vi "HandleObservationSync_003.vi"(8 "error in (no error)":errorcluster, 11 "S4GUI in":refnum<class "S4GUI.lvclass">) -> (0 "error out":errorcluster, 3 "S4GUI out":refnum<class "S4GUI.lvclass">)   [LabVIEW 2018, in "S4GUI.lvclass"] (continued)
          n1276 = call "Read connection.vi"("error in (no error)"=w3469, "Server in"=w3471) -> ("error out"=w3497:errorcluster, "connection"=w3481:bool, "Server out"=w3498:refnum<class "Acquisition.lvclass">)  [unwired: 7 in]
          n1277 = And(x=w3481, y=w3459) -> (x .and. y?=w3482:bool)
          n1278 = case shown="True" w3482 {
            tunnel: w3498 -> [w3607 w3623]
            tunnel: w3497 -> [w3606 w3622]
            tunnel: [w3607 w3620] -> w3515
            tunnel: [w3606 w3619] -> w3513
            tunnel: [w3603 u32 0 ("New_State")] -> w3488
            tunnel: w3459 -> [w3602 _]
            frame False {
              n1279 = Select(t=u32 2, s=w3602, f=u32 0) -> (s? t:f=w3603:u32)
            }
            frame True {
              n1280 = call-dynamic "Read Channel.vi"("error in (no error)"=w3622, "Acquisition in"=w3623) -> ("error out"=w3615:errorcluster, "Channel.lvclass"=w3614:refnum<class "Channel.lvclass">, "Acquisition out"=w3621:refnum<class "Acquisition.lvclass">)  [unwired: 7 in]
              n1281 = call-dynamic "Read State Machine.vi"("error in (no error)"=w3615, "Device in"=w3614) -> ("error out"=w3616:errorcluster, "State Machine.lvclass"=w3618:refnum<class "State Machine.lvclass">, "Device out"=w3612:refnum<class "Channel.lvclass">)  [unwired: 7 in]
              n1282 = call "Next State.vi"("error in (no error)"=w3616, "New_State"=50, "State Machine in"=w3618) -> ("error out"=w3609:errorcluster, "State Machine out"=w3610:refnum<class "State Machine.lvclass">)  [unwired: 7 in]
              n1283 = call-dynamic "Write State Machine.vi"("error in (no error)"=w3609, "State Machine.lvclass"=w3610, "Device in"=w3612) -> ("error out"=w3611:errorcluster, "Device out"=w3613:refnum<class "Channel.lvclass">)  [unwired: 7 in]
              n1284 = call-dynamic "Write Channel.vi"("error in (no error)"=w3611, "Channel.lvclass"=w3613, "Acquisition in"=w3621) -> ("error out"=w3619:errorcluster, "Acquisition out"=w3620:refnum<class "Acquisition.lvclass">)  [unwired: 7 in]
            }
          }
          n1285 = call "Write AcquisitionB.vi"("error in (no error)"=w3513, "Acquisition.lvclass"=w3515, "S4ACS_GUI in"=w3514) -> ("error out"=w3509:errorcluster, "S4ACS_GUI out"=w3508:refnum<class "S4GUI.lvclass">)  [unwired: 7 in]
          n1286 = call-dynamic "Read AcquisitionC.vi"("error in (no error)"=w3509, "S4ACS_GUI in"=w3508) -> ("error out"=w3466:errorcluster, "Acquisition.lvclass"=w3468:refnum<class "Acquisition.lvclass">, "S4ACS_GUI out"=w3511:refnum<class "S4GUI.lvclass">)  [unwired: 7 in]
          n1287 = call-dynamic "Read enabled.vi"("error in (no error)"=w3466, "Server in"=w3468) -> ("error out"=w3465:errorcluster, "enabled"=w3458:bool, "Server out"=w3467:refnum<class "Acquisition.lvclass">)  [unwired: 7 in]
          n1288 = call "Read connection.vi"("error in (no error)"=w3465, "Server in"=w3467) -> ("error out"=w3495:errorcluster, "connection"=w3478:bool, "Server out"=w3496:refnum<class "Acquisition.lvclass">)  [unwired: 7 in]
          n1289 = And(x=w3478, y=w3458) -> (x .and. y?=w3480:bool)
          n1290 = case shown="True" w3480 {
            tunnel: [w3584 w3593] -> w3512
            tunnel: [w3585 w3592] -> w3510
            tunnel: w3496 -> [w3585 w3590]
            tunnel: w3495 -> [w3584 w3589]
            tunnel: [w3581 u32 0 ("New_State")] -> w3487
            tunnel: w3458 -> [w3580 _]
            frame False {
              n1291 = Select(t=u32 4, s=w3580, f=u32 0) -> (s? t:f=w3581:u32)
            }
            frame True {
              n1292 = call-dynamic "Read Channel.vi"("error in (no error)"=w3589, "Acquisition in"=w3590) -> ("error out"=w3597:errorcluster, "Channel.lvclass"=w3598:refnum<class "Channel.lvclass">, "Acquisition out"=w3591:refnum<class "Acquisition.lvclass">)  [unwired: 7 in]
              n1293 = call-dynamic "Read State Machine.vi"("error in (no error)"=w3597, "Device in"=w3598) -> ("error out"=w3596:errorcluster, "State Machine.lvclass"=w3594:refnum<class "State Machine.lvclass">, "Device out"=w3600:refnum<class "Channel.lvclass">)  [unwired: 7 in]
              n1294 = call "Next State.vi"("error in (no error)"=w3596, "New_State"=50, "State Machine in"=w3594) -> ("error out"=w3588:errorcluster, "State Machine out"=w3587:refnum<class "State Machine.lvclass">)  [unwired: 7 in]
              n1295 = call-dynamic "Write State Machine.vi"("error in (no error)"=w3588, "State Machine.lvclass"=w3587, "Device in"=w3600) -> ("error out"=w3601:errorcluster, "Device out"=w3599:refnum<class "Channel.lvclass">)  [unwired: 7 in]
              n1296 = call-dynamic "Write Channel.vi"("error in (no error)"=w3601, "Channel.lvclass"=w3599, "Acquisition in"=w3591) -> ("error out"=w3593:errorcluster, "Acquisition out"=w3592:refnum<class "Acquisition.lvclass">)  [unwired: 7 in]
            }
          }
          n1297 = call-dynamic "Write AcquisitionC.vi"("error in (no error)"=w3512, "Acquisition.lvclass"=w3510, "S4ACS_GUI in"=w3511) -> ("error out"=w3506:errorcluster, "S4ACS_GUI out"=w3505:refnum<class "S4GUI.lvclass">)  [unwired: 7 in]
          n1298 = call-dynamic "Read AcquisitionD.vi"("error in (no error)"=w3506, "S4ACS_GUI in"=w3505) -> ("error out"=w3462:errorcluster, "Acquisition.lvclass"=w3464:refnum<class "Acquisition.lvclass">, "S4ACS_GUI out"=w3504:refnum<class "S4GUI.lvclass">)  [unwired: 7 in]
          n1299 = call-dynamic "Read enabled.vi"("error in (no error)"=w3462, "Server in"=w3464) -> ("error out"=w3461:errorcluster, "enabled"=w3457:bool, "Server out"=w3463:refnum<class "Acquisition.lvclass">)  [unwired: 7 in]
          n1300 = call "Read connection.vi"("error in (no error)"=w3461, "Server in"=w3463) -> ("error out"=w3493:errorcluster, "connection"=w3477:bool, "Server out"=w3494:refnum<class "Acquisition.lvclass">)  [unwired: 7 in]
          n1301 = And(x=w3477, y=w3457) -> (x .and. y?=w3479:bool)
          n1302 = case shown="True" w3479 {
            tunnel: w3493 -> [w3562 w3579]
            tunnel: [w3562 w3578] -> w3507
            tunnel: w3494 -> [w3563 w3569]
            tunnel: [w3563 w3567] -> w3503
            tunnel: [w3559 u32 0 ("New_State")] -> w3486
            tunnel: w3457 -> [w3558 _]
            frame False {
              n1303 = Select(t=u32 8, s=w3558, f=u32 0) -> (s? t:f=w3559:u32)
            }
            frame True {
              n1304 = call-dynamic "Read Channel.vi"("error in (no error)"=w3579, "Acquisition in"=w3569) -> ("error out"=w3574:errorcluster, "Channel.lvclass"=w3573:refnum<class "Channel.lvclass">, "Acquisition out"=w3568:refnum<class "Acquisition.lvclass">)  [unwired: 7 in]
              n1305 = call-dynamic "Read State Machine.vi"("error in (no error)"=w3574, "Device in"=w3573) -> ("error out"=w3575:errorcluster, "State Machine.lvclass"=w3577:refnum<class "State Machine.lvclass">, "Device out"=w3571:refnum<class "Channel.lvclass">)  [unwired: 7 in]
              n1306 = call "Next State.vi"("error in (no error)"=w3575, "New_State"=50, "State Machine in"=w3577) -> ("error out"=w3565:errorcluster, "State Machine out"=w3566:refnum<class "State Machine.lvclass">)  [unwired: 7 in]
              n1307 = call-dynamic "Write State Machine.vi"("error in (no error)"=w3565, "State Machine.lvclass"=w3566, "Device in"=w3571) -> ("error out"=w3570:errorcluster, "Device out"=w3572:refnum<class "Channel.lvclass">)  [unwired: 7 in]
              n1308 = call-dynamic "Write Channel.vi"("error in (no error)"=w3570, "Channel.lvclass"=w3572, "Acquisition in"=w3568) -> ("error out"=w3578:errorcluster, "Acquisition out"=w3567:refnum<class "Acquisition.lvclass">)  [unwired: 7 in]
            }
          }
          n1309 = call-dynamic "Write AcquisitionD.vi"("error in (no error)"=w3507, "Acquisition.lvclass"=w3503, "S4ACS_GUI in"=w3504) -> ("error out"=w3502:errorcluster, "S4ACS_GUI out"=w3501:refnum<class "S4GUI.lvclass">)  [unwired: 7 in]
          n1310 = Compound Arithmetic op=ADD(w3489, w3488, w3487, w3486) -> (w3490:u32)
          n1311 = case shown="0, Default" w3490 {
            tunnel: w3485 -> [w3527 _ _ _ _ _ _ _ _ _ _ _ _ _ _ _]
            tunnel: [w3526 u32 1 ("Obs_state") u32 1 ("Obs_state") u32 1 ("Obs_state") u32 1 ("Obs_state") u32 1 ("Obs_state") u32 1 ("Obs_state") u32 1 ("Obs_state") u32 1 ("Obs_state") u32 1 ("Obs_state") u32 1 ("Obs_state") u32 1 ("Obs_state") u32 1 ("Obs_state") u32 1 ("Obs_state") u32 1 ("Obs_state") u32 1 ("Obs_state")] -> w3491
            tunnel: ["" ("Error Msg") "ERROR: Lost channel 1 connection... - HandleObservationSync.vi state 323" ("Error Msg") "ERROR: Lost channel 2 connection...- HandleObservationSync.vi state 323" ("Error Msg") "ERROR: Lost channels 1 and 2 connection...- HandleObservationSync.vi state 323" ("Error Msg") "ERROR: Lost channel 3 connection...- HandleObservationSync.vi state 323" ("Error Msg") "ERROR: Lost channels 1 and  3 connection...- HandleObservationSync.vi state 323" ("Error Msg") "ERROR:  Lost channels 2 and  3 connection...- HandleObservationSync.vi state 323" ("Error Msg") "ERROR:  Lost channels 1, 2 and  3 connection...- HandleObservationSync.vi state 323" ("Error Msg") "ERROR: Lost channel 4 connection...- HandleObservationSync.vi state 323" ("Error Msg") "ERROR:  Lost channels 1 and 4 connection...- HandleObservationSync.vi state 323" ("Error Msg") "ERROR:  Lost channels 2 and 4 connection...- HandleObservationSync.vi state 323" ("Error Msg") "ERROR: Lost channels 1, 2 and 4 connection...- HandleObservationSync.vi state 323" ("Error Msg") "ERROR: Lost channels 3 and 4 connection...- HandleObservationSync.vi state 323" ("Error Msg") "ERROR: Lost channels 1, 3 and 4 connection...- HandleObservationSync.vi state 323" ("Error Msg") "ERROR: Lost channels 2, 3 and 4 connection...- HandleObservationSync.vi state 323" ("Error Msg") "ERROR: Lost channels 1, 2, 3 and 4 connection...- HandleObservationSync.vi state 323" ("Error Msg")] -> w3492
            frame 0, Default {
              n1312 = Increment(x=w3527) -> (x+1=w3526:u32)
              n1313 = Tick Count (ms)() -> (millisecond timer value=w3524:u32)
              n1314 = local write "time1"(w3524) -> ()
            }
            frame 1 {
            }
            frame 2 {
            }
            frame 3 {
            }
            frame 4 {
            }
            frame 5 {
            }
            frame 6 {
            }
            frame 7 {
            }
            frame 8 {
            }
            frame 9 {
            }
            frame 10 {
            }
            frame 11 {
            }
            frame 12 {
            }
            frame 13 {
            }
            frame 14 {
            }
            frame 15 {
            }
          }
          n1315 = Bundle By Name(cluster=w3501, "Obs_state"=w3491, "Error Msg"=w3492) -> (w3518:refnum<class "S4GUI.lvclass">)
        }
        frame 324 {
          # "Espera terminar a execução do comando atual \nantes de ir ao proximo passo da Observação."
          n1316 = call-dynamic "Read AcquisitionA.vi"("error in (no error)"=w3699, "S4ACS_GUI in"=w3700) -> ("error out"=w3681:errorcluster, "Acquisition.lvclass"=w3682:refnum<class "Acquisition.lvclass">, "S4ACS_GUI out"=w3702:refnum<class "S4GUI.lvclass">)  [unwired: 7 in]
          n1317 = call "Read connection.vi"("error in (no error)"=w3681, "Server in"=w3682) -> ("error out"=w3680:errorcluster, "connection"=w3679:bool, "Server out"=w3678:refnum<class "Acquisition.lvclass">)  [unwired: 7 in]
          n1318 = case shown="True" w3679 {
            tunnel: w3680 -> [w3811 w3832]
            tunnel: [w3812 w3830] -> w3703
            tunnel: [w3811 w3829] -> w3701
            tunnel: [TRUE w3818] -> w3660
            tunnel: w3678 -> [w3812 w3821]
            tunnel: [FALSE w3813] -> w3658
            frame False {
            }
            frame True {
              n1319 = call-dynamic "Read Channel.vi"("error in (no error)"=w3832, "Acquisition in"=w3821) -> ("error out"=w3815:errorcluster, "Channel.lvclass"=w3817:refnum<class "Channel.lvclass">, "Acquisition out"=w3831:refnum<class "Acquisition.lvclass">)  [unwired: 7 in]
              n1320 = call-dynamic "Read wait_expose.vi"("error in (no error)"=w3815, "Channel in"=w3817) -> ("error out"=w3814:errorcluster, "wait_expose"=w3813:bool, "Channel out"=w3816:refnum<class "Channel.lvclass">)  [unwired: 7 in]
              n1321 = call-dynamic "Read State Machine.vi"("error in (no error)"=w3814, "Device in"=w3816) -> ("error out"=w3823:errorcluster, "State Machine.lvclass"=w3825:refnum<class "State Machine.lvclass">, "Device out"=w3827:refnum<class "Channel.lvclass">)  [unwired: 7 in]
              n1322 = call-dynamic "Read State.vi"("error in (no error)"=w3823, "State Machine in"=w3825) -> ("error out"=w3822:errorcluster, "State"=w3819:i32, "State Machine out"=w3824:refnum<class "State Machine.lvclass">)  [unwired: 7 in]
              n1323 = Greater?(x=w3819, y=53 ("x")) -> (0:w3818:bool)
              n1324 = call-dynamic "Write State Machine.vi"("error in (no error)"=w3822, "State Machine.lvclass"=w3824, "Device in"=w3827) -> ("error out"=w3826:errorcluster, "Device out"=w3828:refnum<class "Channel.lvclass">)  [unwired: 7 in]
              n1325 = call-dynamic "Write Channel.vi"("error in (no error)"=w3826, "Channel.lvclass"=w3828, "Acquisition in"=w3831) -> ("error out"=w3829:errorcluster, "Acquisition out"=w3830:refnum<class "Acquisition.lvclass">)  [unwired: 7 in]
            }
          }
          n1326 = call-dynamic "Write AcquisitionA.vi"("error in (no error)"=w3701, "Acquisition.lvclass"=w3703, "S4ACS_GUI in"=w3702) -> ("error out"=w3696:errorcluster, "S4ACS_GUI out"=w3695:refnum<class "S4GUI.lvclass">)  [unwired: 7 in]
          n1327 = call "Read AcquisitionB.vi"("error in (no error)"=w3696, "S4ACS_GUI in"=w3695) -> ("error out"=w3673:errorcluster, "Acquisition.lvclass"=w3677:refnum<class "Acquisition.lvclass">, "S4ACS_GUI out"=w3697:refnum<class "S4GUI.lvclass">)  [unwired: 7 in]
          n1328 = call "Read connection.vi"("error in (no error)"=w3673, "Server in"=w3677) -> ("error out"=w3674:errorcluster, "connection"=w3675:bool, "Server out"=w3676:refnum<class "Acquisition.lvclass">)  [unwired: 7 in]
          n1329 = case shown="True" w3675 {
            tunnel: w3674 -> [w3787 w3800]
            tunnel: w3676 -> [w3788 w3799]
            tunnel: [TRUE w3794] -> w3662
            tunnel: [w3787 w3798] -> w3694
            tunnel: [w3788 w3797] -> w3693
            tunnel: [FALSE w3789] -> w3657
            frame False {
            }
            frame True {
              n1330 = call-dynamic "Read Channel.vi"("error in (no error)"=w3800, "Acquisition in"=w3799) -> ("error out"=w3791:errorcluster, "Channel.lvclass"=w3793:refnum<class "Channel.lvclass">, "Acquisition out"=w3801:refnum<class "Acquisition.lvclass">)  [unwired: 7 in]
              n1331 = call-dynamic "Read wait_expose.vi"("error in (no error)"=w3791, "Channel in"=w3793) -> ("error out"=w3790:errorcluster, "wait_expose"=w3789:bool, "Channel out"=w3792:refnum<class "Channel.lvclass">)  [unwired: 7 in]
              n1332 = call-dynamic "Read State Machine.vi"("error in (no error)"=w3790, "Device in"=w3792) -> ("error out"=w3807:errorcluster, "State Machine.lvclass"=w3805:refnum<class "State Machine.lvclass">, "Device out"=w3803:refnum<class "Channel.lvclass">)  [unwired: 7 in]
              n1333 = call-dynamic "Read State.vi"("error in (no error)"=w3807, "State Machine in"=w3805) -> ("error out"=w3808:errorcluster, "State"=w3796:i32, "State Machine out"=w3806:refnum<class "State Machine.lvclass">)  [unwired: 7 in]
              n1334 = Greater?(x=w3796, y=53 ("x")) -> (0:w3794:bool)
              n1335 = call-dynamic "Write State Machine.vi"("error in (no error)"=w3808, "State Machine.lvclass"=w3806, "Device in"=w3803) -> ("error out"=w3804:errorcluster, "Device out"=w3802:refnum<class "Channel.lvclass">)  [unwired: 7 in]
              n1336 = call-dynamic "Write Channel.vi"("error in (no error)"=w3804, "Channel.lvclass"=w3802, "Acquisition in"=w3801) -> ("error out"=w3798:errorcluster, "Acquisition out"=w3797:refnum<class "Acquisition.lvclass">)  [unwired: 7 in]
            }
          }
          n1337 = call "Write AcquisitionB.vi"("error in (no error)"=w3694, "Acquisition.lvclass"=w3693, "S4ACS_GUI in"=w3697) -> ("error out"=w3686:errorcluster, "S4ACS_GUI out"=w3685:refnum<class "S4GUI.lvclass">)  [unwired: 7 in]
          n1338 = call-dynamic "Read AcquisitionC.vi"("error in (no error)"=w3686, "S4ACS_GUI in"=w3685) -> ("error out"=w3669:errorcluster, "Acquisition.lvclass"=w3672:refnum<class "Acquisition.lvclass">, "S4ACS_GUI out"=w3688:refnum<class "S4GUI.lvclass">)  [unwired: 7 in]
          n1339 = call "Read connection.vi"("error in (no error)"=w3669, "Server in"=w3672) -> ("error out"=w3668:errorcluster, "connection"=w3670:bool, "Server out"=w3671:refnum<class "Acquisition.lvclass">)  [unwired: 7 in]
          n1340 = case shown="True" w3670 {
            tunnel: [w3763 w3777] -> w3689
            tunnel: [w3764 w3776] -> w3687
            tunnel: w3668 -> [w3763 w3773]
            tunnel: w3671 -> [w3764 w3774]
            tunnel: [TRUE w3770] -> w3661
            tunnel: [FALSE w3765] -> w3656
            frame False {
            }
            frame True {
              n1341 = call-dynamic "Read Channel.vi"("error in (no error)"=w3773, "Acquisition in"=w3774) -> ("error out"=w3767:errorcluster, "Channel.lvclass"=w3769:refnum<class "Channel.lvclass">, "Acquisition out"=w3775:refnum<class "Acquisition.lvclass">)  [unwired: 7 in]
              n1342 = call-dynamic "Read wait_expose.vi"("error in (no error)"=w3767, "Channel in"=w3769) -> ("error out"=w3766:errorcluster, "wait_expose"=w3765:bool, "Channel out"=w3768:refnum<class "Channel.lvclass">)  [unwired: 7 in]
              n1343 = call-dynamic "Read State Machine.vi"("error in (no error)"=w3766, "Device in"=w3768) -> ("error out"=w3783:errorcluster, "State Machine.lvclass"=w3781:refnum<class "State Machine.lvclass">, "Device out"=w3779:refnum<class "Channel.lvclass">)  [unwired: 7 in]
              n1344 = call-dynamic "Read State.vi"("error in (no error)"=w3783, "State Machine in"=w3781) -> ("error out"=w3784:errorcluster, "State"=w3771:i32, "State Machine out"=w3782:refnum<class "State Machine.lvclass">)  [unwired: 7 in]
              n1345 = Greater?(x=w3771, y=53 ("x")) -> (0:w3770:bool)
              n1346 = call-dynamic "Write State Machine.vi"("error in (no error)"=w3784, "State Machine.lvclass"=w3782, "Device in"=w3779) -> ("error out"=w3780:errorcluster, "Device out"=w3778:refnum<class "Channel.lvclass">)  [unwired: 7 in]
              n1347 = call-dynamic "Write Channel.vi"("error in (no error)"=w3780, "Channel.lvclass"=w3778, "Acquisition in"=w3775) -> ("error out"=w3777:errorcluster, "Acquisition out"=w3776:refnum<class "Acquisition.lvclass">)  [unwired: 7 in]
            }
          }
          n1348 = call-dynamic "Write AcquisitionC.vi"("error in (no error)"=w3689, "Acquisition.lvclass"=w3687, "S4ACS_GUI in"=w3688) -> ("error out"=w3683:errorcluster, "S4ACS_GUI out"=w3684:refnum<class "S4GUI.lvclass">)  [unwired: 7 in]
          n1349 = call-dynamic "Read AcquisitionD.vi"("error in (no error)"=w3683, "S4ACS_GUI in"=w3684) -> ("error out"=w3664:errorcluster, "Acquisition.lvclass"=w3667:refnum<class "Acquisition.lvclass">, "S4ACS_GUI out"=w3690:refnum<class "S4GUI.lvclass">)  [unwired: 7 in]
          n1350 = call "Read connection.vi"("error in (no error)"=w3664, "Server in"=w3667) -> ("error out"=w3663:errorcluster, "connection"=w3665:bool, "Server out"=w3666:refnum<class "Acquisition.lvclass">)  [unwired: 7 in]
          n1351 = case shown="True" w3665 {
            tunnel: [w3740 w3760] -> w3692
            tunnel: [w3739 w3759] -> w3691
            tunnel: w3666 -> [w3740 w3758]
            tunnel: w3663 -> [w3739 w3757]
            tunnel: [TRUE w3746] -> w3659
            tunnel: [FALSE w3741] -> w3655
            frame False {
            }
            frame True {
              n1352 = call-dynamic "Read Channel.vi"("error in (no error)"=w3757, "Acquisition in"=w3758) -> ("error out"=w3743:errorcluster, "Channel.lvclass"=w3745:refnum<class "Channel.lvclass">, "Acquisition out"=w3756:refnum<class "Acquisition.lvclass">)  [unwired: 7 in]
              n1353 = call-dynamic "Read wait_expose.vi"("error in (no error)"=w3743, "Channel in"=w3745) -> ("error out"=w3742:errorcluster, "wait_expose"=w3741:bool, "Channel out"=w3744:refnum<class "Channel.lvclass">)  [unwired: 7 in]
              n1354 = call-dynamic "Read State Machine.vi"("error in (no error)"=w3742, "Device in"=w3744) -> ("error out"=w3750:errorcluster, "State Machine.lvclass"=w3752:refnum<class "State Machine.lvclass">, "Device out"=w3754:refnum<class "Channel.lvclass">)  [unwired: 7 in]
              n1355 = call-dynamic "Read State.vi"("error in (no error)"=w3750, "State Machine in"=w3752) -> ("error out"=w3749:errorcluster, "State"=w3747:i32, "State Machine out"=w3751:refnum<class "State Machine.lvclass">)  [unwired: 7 in]
              n1356 = Greater?(x=w3747, y=53 ("x")) -> (0:w3746:bool)
              n1357 = call-dynamic "Write State Machine.vi"("error in (no error)"=w3749, "State Machine.lvclass"=w3751, "Device in"=w3754) -> ("error out"=w3753:errorcluster, "Device out"=w3755:refnum<class "Channel.lvclass">)  [unwired: 7 in]
              n1358 = call-dynamic "Write Channel.vi"("error in (no error)"=w3753, "Channel.lvclass"=w3755, "Acquisition in"=w3756) -> ("error out"=w3759:errorcluster, "Acquisition out"=w3760:refnum<class "Acquisition.lvclass">)  [unwired: 7 in]
            }
          }
          n1359 = call-dynamic "Write AcquisitionD.vi"("error in (no error)"=w3691, "Acquisition.lvclass"=w3692, "S4ACS_GUI in"=w3690) -> ("error out"=w3647:errorcluster, "S4ACS_GUI out"=w3650:refnum<class "S4GUI.lvclass">)  [unwired: 7 in]
          n1360 = Compound Arithmetic op=AND(w3660, w3662, w3661, w3659) -> (w3654:bool)
          n1361 = Compound Arithmetic op=OR(w3658, w3657, w3656, w3655) -> (w3652:bool)
          n1362 = call-dynamic "VerifErrors.vi"("error in (no error)"=w3647, "S4GUI in"=w3650) -> ("error out"=w3646:errorcluster, "Error value"=w3649:u32, "S4GUI out"=w3648:refnum<class "S4GUI.lvclass">)  [unwired: 7 in]
          n1363 = case shown="False" w3654 {
            tunnel: w3648 -> [w3706 w3736]
            tunnel: [w3712 w3735] -> w3651
            tunnel: w3653 -> [_ w3734]
            tunnel: w3652 -> [_ w3730]
            tunnel: w3649 -> [w3704 _]
            frame False {
              # "Aguardando iniciar exposição por 5s"
              n1364 = Tick Count (ms)() -> (millisecond timer value=w3711:u32)
              n1365 = local read "time1"() -> (w3705:u32)
              n1366 = Subtract(x=w3711, y=w3705) -> (x-y=w3708:u32)
              n1367 = To Double Precision Float(number=w3708) -> (double precision float=w3710:dbl)
              n1368 = Less?(x=5000.0 ("y"), y=w3710) -> (x < y?=w3709:bool)
              n1369 = case shown="False" w3709 {
                tunnel: w3706 -> [w3715 w3728]
                tunnel: [w3713 w3727] -> w3712
                tunnel: w3704 -> [w3714 _]
                frame False {
                  n1370 = case shown="1..15" w3714 {
                    selector: w3714 -> [_ w3723]
                    tunnel: [w3716 w3718] -> w3713
                    tunnel: w3715 -> [w3716 w3724]
                    frame 0, Default {
                    }
                    frame 1..15 {
                      n1371 = Number To Decimal String(number=w3723) -> (decimal integer string=w3720:string)  [unwired: 1 in]
                      n1372 = Concatenate Strings("CHANNEL ERROR <", w3720, ">: Error flag TRUE - see ACS panel.  HandleObservationSync.vi - state 324.") -> (w3722:string)
                      n1373 = Bundle By Name(cluster=w3724, "Obs_state"=u32 1, "Error Msg"=w3722) -> (w3718:refnum<class "S4GUI.lvclass">)
                    }
                  }
                }
                frame True {
                  n1374 = Bundle By Name(cluster=w3728, "Obs_state"=u32 1, "Error Msg"="ERROR: Acquisition Timeout. HandleObservationSync.vi - state 324.") -> (w3727:refnum<class "S4GUI.lvclass">)
                }
              }
            }
            frame True {
              # "327: Verifica incremento de ciclo."
              # "Iniciou aquisição..."
              n1375 = Increment(x=w3734) -> (x+1=w3731:u32)
              n1376 = Select(t=u32 327, s=w3730, f=w3731) -> (s? t:f=w3729:u32)
              n1377 = Tick Count (ms)() -> (millisecond timer value=w3733:u32)
              n1378 = Bundle By Name(cluster=w3736, "Obs_state"=w3729) -> (w3735:refnum<class "S4GUI.lvclass">)
              n1379 = local write "time307"(w3733) -> ()
            }
          }
          n1380 = Bundle By Name(cluster=w3651, "mode EXPOSE"=w3652) -> (w3698:refnum<class "S4GUI.lvclass">)
        }
        frame 325 {
          n1381 = Unbundle By Name(w3842) -> ("mode EXPOSE"=w3841:bool)
          n1382 = case shown="True" w3841 {
            tunnel: w3842 -> [w3895 w3962]
            tunnel: w3847 -> [w3894 w3961]
            tunnel: [w3893 w3959] -> w3846
            tunnel: [w3892 w3960] -> w3845
            tunnel: [w3891 w3958] -> w3835
            tunnel: w3843 -> [w3883 w3958]
            tunnel: [w3882 w3923] -> w3840
            tunnel: [w3882 w3922] -> w3839
            tunnel: [w3882 w3921] -> w3838
            tunnel: [w3882 w3920] -> w3837
            frame False {
              w3882 = 0
              n1383 = call-dynamic "Read Sync Box.lvclass.vi"("error in (no error)"=w3894, "SPARC4_AC in"=w3895) -> ("error out"=w3888:errorcluster, "Sync Box.lvclass"=w3890:refnum<class "Sync Box.lvclass">, "SPARC4_AC out"=w3885:refnum<class "S4GUI.lvclass">)  [unwired: 7 in]
              n1384 = call "Read connection.vi"("error in (no error)"=w3888, "Server in"=w3890) -> ("error out"=w3887:errorcluster, "connection"=w3886:bool, "Server out"=w3889:refnum<class "Sync Box.lvclass">)  [unwired: 7 in]
              n1385 = case shown="True" w3886 {
                tunnel: w3887 -> [w3901 w3919]
                tunnel: [w3902 w3917] -> w3897
                tunnel: [w3901 w3904] -> w3896
                tunnel: w3883 -> [w3898 w3903]
                tunnel: [w3900 w3903] -> w3891
                tunnel: w3889 -> [w3902 w3908]
                tunnel: w3885 -> [w3899 w3905]
                tunnel: [w3899 w3905] -> w3884
                frame False {
                  n1386 = Increment(x=w3898) -> (x+1=w3900:u32)
                }
                frame True {
                  # "Envia comando FIRE para o SyncBox"
                  n1387 = call-dynamic "Read Trigger.lvclass.vi"("error in (no error)"=w3919, "Sync Box in"=w3908) -> ("error out"=w3913:errorcluster, "Trigger.lvclass"=w3912:refnum<class "Trigger.lvclass">, "Sync Box out"=w3918:refnum<class "Sync Box.lvclass">)  [unwired: 7 in]
                  n1388 = call-dynamic "Read State Machine.vi"("error in (no error)"=w3913, "Device in"=w3912) -> ("error out"=w3914:errorcluster, "State Machine.lvclass"=w3916:refnum<class "State Machine.lvclass">, "Device out"=w3910:refnum<class "Trigger.lvclass">)  [unwired: 7 in]
                  n1389 = call "Next State.vi"("error in (no error)"=w3914, "New_State"=40, "State Machine in"=w3916) -> ("error out"=w3906:errorcluster, "State Machine out"=w3907:refnum<class "State Machine.lvclass">)  [unwired: 7 in]
                  n1390 = call-dynamic "Write State Machine.vi"("error in (no error)"=w3906, "State Machine.lvclass"=w3907, "Device in"=w3910) -> ("error out"=w3909:errorcluster, "Device out"=w3911:refnum<class "Trigger.lvclass">)  [unwired: 7 in]
                  n1391 = call-dynamic "Write Trigger.lvclass.vi"("error in (no error)"=w3909, "Trigger.lvclass"=w3911, "Sync Box in"=w3918) -> ("error out"=w3904:errorcluster, "Sync Box out"=w3917:refnum<class "Sync Box.lvclass">)  [unwired: 7 in]
                }
              }
              n1392 = call-dynamic "Write Sync Box.lvclass.vi"("error in (no error)"=w3896, "Sync Box.lvclass"=w3897, "SPARC4_AC in"=w3884) -> ("error out"=w3893:errorcluster, "SPARC4_AC out"=w3892:refnum<class "S4GUI.lvclass">)  [unwired: 7 in]
            }
            frame True {
              # "Envia comando EXPOSE para os canais ativos"
              n1393 = call-dynamic "Read AcquisitionA.vi"("error in (no error)"=w3961, "S4ACS_GUI in"=w3962) -> ("error out"=w3955:errorcluster, "Acquisition.lvclass"=w3957:refnum<class "Acquisition.lvclass">, "S4ACS_GUI out"=w3981:refnum<class "S4GUI.lvclass">)  [unwired: 7 in]
              n1394 = call-dynamic "Read enabled.vi"("error in (no error)"=w3955, "Server in"=w3957) -> ("error out"=w3954:errorcluster, "enabled"=w3927:bool, "Server out"=w3956:refnum<class "Acquisition.lvclass">)  [unwired: 7 in]
              n1395 = call "Read connection.vi"("error in (no error)"=w3954, "Server in"=w3956) -> ("error out"=w3963:errorcluster, "connection"=w3952:bool, "Server out"=w3964:refnum<class "Acquisition.lvclass">)  [unwired: 7 in]
              n1396 = And(x=w3952, y=w3927) -> (x .and. y?=w3953:bool)
              n1397 = case shown="True" w3953 {
                tunnel: w3964 -> [w4054 w4070]
                tunnel: w3963 -> [w4053 w4069]
                tunnel: [w4054 w4067] -> w3982
                tunnel: [w4053 w4066] -> w3980
                tunnel: [w4049 0] -> w3923
                tunnel: w3927 -> [w4050 _]
                frame False {
                  n1398 = Select(t=1, s=w4050, f=0) -> (s? t:f=w4049:i32)
                }
                frame True {
                  n1399 = call-dynamic "Read Channel.vi"("error in (no error)"=w4069, "Acquisition in"=w4070) -> ("error out"=w4062:errorcluster, "Channel.lvclass"=w4061:refnum<class "Channel.lvclass">, "Acquisition out"=w4068:refnum<class "Acquisition.lvclass">)  [unwired: 7 in]
                  n1400 = call-dynamic "Read State Machine.vi"("error in (no error)"=w4062, "Device in"=w4061) -> ("error out"=w4063:errorcluster, "State Machine.lvclass"=w4065:refnum<class "State Machine.lvclass">, "Device out"=w4059:refnum<class "Channel.lvclass">)  [unwired: 7 in]
                  n1401 = call "Next State.vi"("error in (no error)"=w4063, "New_State"=50, "State Machine in"=w4065) -> ("error out"=w4056:errorcluster, "State Machine out"=w4057:refnum<class "State Machine.lvclass">)  [unwired: 7 in]
                  n1402 = call-dynamic "Write State Machine.vi"("error in (no error)"=w4056, "State Machine.lvclass"=w4057, "Device in"=w4059) -> ("error out"=w4058:errorcluster, "Device out"=w4060:refnum<class "Channel.lvclass">)  [unwired: 7 in]
                  n1403 = call-dynamic "Write Channel.vi"("error in (no error)"=w4058, "Channel.lvclass"=w4060, "Acquisition in"=w4068) -> ("error out"=w4066:errorcluster, "Acquisition out"=w4067:refnum<class "Acquisition.lvclass">)  [unwired: 7 in]
                }
              }
              n1404 = call-dynamic "Write AcquisitionA.vi"("error in (no error)"=w3980, "Acquisition.lvclass"=w3982, "S4ACS_GUI in"=w3981) -> ("error out"=w3978:errorcluster, "S4ACS_GUI out"=w3979:refnum<class "S4GUI.lvclass">)  [unwired: 7 in]
              n1405 = call "Read AcquisitionB.vi"("error in (no error)"=w3978, "S4ACS_GUI in"=w3979) -> ("error out"=w3946:errorcluster, "Acquisition.lvclass"=w3948:refnum<class "Acquisition.lvclass">, "S4ACS_GUI out"=w3976:refnum<class "S4GUI.lvclass">)  [unwired: 7 in]
              n1406 = call-dynamic "Read enabled.vi"("error in (no error)"=w3946, "Server in"=w3948) -> ("error out"=w3950:errorcluster, "enabled"=w3926:bool, "Server out"=w3951:refnum<class "Acquisition.lvclass">)  [unwired: 7 in]
              n1407 = call "Read connection.vi"("error in (no error)"=w3950, "Server in"=w3951) -> ("error out"=w3945:errorcluster, "connection"=w3949:bool, "Server out"=w3947:refnum<class "Acquisition.lvclass">)  [unwired: 7 in]
              n1408 = And(x=w3949, y=w3926) -> (x .and. y?=w3944:bool)
              n1409 = case shown="False" w3944 {
                tunnel: w3947 -> [w4032 w4048]
                tunnel: w3945 -> [w4031 w4047]
                tunnel: [w4032 w4045] -> w3977
                tunnel: [w4031 w4044] -> w3975
                tunnel: [w4028 0] -> w3922
                tunnel: w3926 -> [w4027 _]
                frame False {
                  n1410 = Select(t=2, s=w4027, f=0) -> (s? t:f=w4028:i32)
                }
                frame True {
                  n1411 = call-dynamic "Read Channel.vi"("error in (no error)"=w4047, "Acquisition in"=w4048) -> ("error out"=w4040:errorcluster, "Channel.lvclass"=w4039:refnum<class "Channel.lvclass">, "Acquisition out"=w4046:refnum<class "Acquisition.lvclass">)  [unwired: 7 in]
                  n1412 = call-dynamic "Read State Machine.vi"("error in (no error)"=w4040, "Device in"=w4039) -> ("error out"=w4041:errorcluster, "State Machine.lvclass"=w4043:refnum<class "State Machine.lvclass">, "Device out"=w4037:refnum<class "Channel.lvclass">)  [unwired: 7 in]
                  n1413 = call "Next State.vi"("error in (no error)"=w4041, "New_State"=50, "State Machine in"=w4043) -> ("error out"=w4034:errorcluster, "State Machine out"=w4035:refnum<class "State Machine.lvclass">)  [unwired: 7 in]
                  n1414 = call-dynamic "Write State Machine.vi"("error in (no error)"=w4034, "State Machine.lvclass"=w4035, "Device in"=w4037) -> ("error out"=w4036:errorcluster, "Device out"=w4038:refnum<class "Channel.lvclass">)  [unwired: 7 in]
                  n1415 = call-dynamic "Write Channel.vi"("error in (no error)"=w4036, "Channel.lvclass"=w4038, "Acquisition in"=w4046) -> ("error out"=w4044:errorcluster, "Acquisition out"=w4045:refnum<class "Acquisition.lvclass">)  [unwired: 7 in]
                }
              }
              n1416 = call "Write AcquisitionB.vi"("error in (no error)"=w3975, "Acquisition.lvclass"=w3977, "S4ACS_GUI in"=w3976) -> ("error out"=w3971:errorcluster, "S4ACS_GUI out"=w3970:refnum<class "S4GUI.lvclass">)  [unwired: 7 in]
              n1417 = call-dynamic "Read AcquisitionC.vi"("error in (no error)"=w3971, "S4ACS_GUI in"=w3970) -> ("error out"=w3937:errorcluster, "Acquisition.lvclass"=w3938:refnum<class "Acquisition.lvclass">, "S4ACS_GUI out"=w3973:refnum<class "S4GUI.lvclass">)  [unwired: 7 in]
              n1418 = call-dynamic "Read enabled.vi"("error in (no error)"=w3937, "Server in"=w3938) -> ("error out"=w3942:errorcluster, "enabled"=w3925:bool, "Server out"=w3943:refnum<class "Acquisition.lvclass">)  [unwired: 7 in]
              n1419 = call "Read connection.vi"("error in (no error)"=w3942, "Server in"=w3943) -> ("error out"=w3939:errorcluster, "connection"=w3941:bool, "Server out"=w3940:refnum<class "Acquisition.lvclass">)  [unwired: 7 in]
              n1420 = And(x=w3941, y=w3925) -> (x .and. y?=w3936:bool)
              n1421 = case shown="False" w3936 {
                tunnel: [w4009 w4018] -> w3974
                tunnel: [w4010 w4017] -> w3972
                tunnel: w3940 -> [w4010 w4015]
                tunnel: w3939 -> [w4009 w4014]
                tunnel: [w4005 0] -> w3921
                tunnel: w3925 -> [w4006 _]
                frame False {
                  n1422 = Select(t=4, s=w4006, f=0) -> (s? t:f=w4005:i32)
                }
                frame True {
                  n1423 = call-dynamic "Read Channel.vi"("error in (no error)"=w4014, "Acquisition in"=w4015) -> ("error out"=w4022:errorcluster, "Channel.lvclass"=w4023:refnum<class "Channel.lvclass">, "Acquisition out"=w4016:refnum<class "Acquisition.lvclass">)  [unwired: 7 in]
                  n1424 = call-dynamic "Read State Machine.vi"("error in (no error)"=w4022, "Device in"=w4023) -> ("error out"=w4021:errorcluster, "State Machine.lvclass"=w4019:refnum<class "State Machine.lvclass">, "Device out"=w4025:refnum<class "Channel.lvclass">)  [unwired: 7 in]
                  n1425 = call "Next State.vi"("error in (no error)"=w4021, "New_State"=50, "State Machine in"=w4019) -> ("error out"=w4013:errorcluster, "State Machine out"=w4012:refnum<class "State Machine.lvclass">)  [unwired: 7 in]
                  n1426 = call-dynamic "Write State Machine.vi"("error in (no error)"=w4013, "State Machine.lvclass"=w4012, "Device in"=w4025) -> ("error out"=w4026:errorcluster, "Device out"=w4024:refnum<class "Channel.lvclass">)  [unwired: 7 in]
                  n1427 = call-dynamic "Write Channel.vi"("error in (no error)"=w4026, "Channel.lvclass"=w4024, "Acquisition in"=w4016) -> ("error out"=w4018:errorcluster, "Acquisition out"=w4017:refnum<class "Acquisition.lvclass">)  [unwired: 7 in]
                }
              }
              n1428 = call-dynamic "Write AcquisitionC.vi"("error in (no error)"=w3974, "Acquisition.lvclass"=w3972, "S4ACS_GUI in"=w3973) -> ("error out"=w3968:errorcluster, "S4ACS_GUI out"=w3967:refnum<class "S4GUI.lvclass">)  [unwired: 7 in]
              n1429 = call-dynamic "Read AcquisitionD.vi"("error in (no error)"=w3968, "S4ACS_GUI in"=w3967) -> ("error out"=w3929:errorcluster, "Acquisition.lvclass"=w3930:refnum<class "Acquisition.lvclass">, "S4ACS_GUI out"=w3966:refnum<class "S4GUI.lvclass">)  [unwired: 7 in]
              n1430 = call-dynamic "Read enabled.vi"("error in (no error)"=w3929, "Server in"=w3930) -> ("error out"=w3934:errorcluster, "enabled"=w3924:bool, "Server out"=w3935:refnum<class "Acquisition.lvclass">)  [unwired: 7 in]
              n1431 = call "Read connection.vi"("error in (no error)"=w3934, "Server in"=w3935) -> ("error out"=w3932:errorcluster, "connection"=w3933:bool, "Server out"=w3931:refnum<class "Acquisition.lvclass">)  [unwired: 7 in]
              n1432 = And(x=w3933, y=w3924) -> (x .and. y?=w3928:bool)
              n1433 = case shown="False" w3928 {
                tunnel: w3932 -> [w3987 w4004]
                tunnel: [w3987 w4003] -> w3969
                tunnel: w3931 -> [w3988 w3994]
                tunnel: [w3988 w3992] -> w3965
                tunnel: [w3983 0] -> w3920
                tunnel: w3924 -> [w3984 _]
                frame False {
                  n1434 = Select(t=8, s=w3984, f=0) -> (s? t:f=w3983:i32)
                }
                frame True {
                  n1435 = call-dynamic "Read Channel.vi"("error in (no error)"=w4004, "Acquisition in"=w3994) -> ("error out"=w3999:errorcluster, "Channel.lvclass"=w3998:refnum<class "Channel.lvclass">, "Acquisition out"=w3993:refnum<class "Acquisition.lvclass">)  [unwired: 7 in]
                  n1436 = call-dynamic "Read State Machine.vi"("error in (no error)"=w3999, "Device in"=w3998) -> ("error out"=w4000:errorcluster, "State Machine.lvclass"=w4002:refnum<class "State Machine.lvclass">, "Device out"=w3996:refnum<class "Channel.lvclass">)  [unwired: 7 in]
                  n1437 = call "Next State.vi"("error in (no error)"=w4000, "New_State"=50, "State Machine in"=w4002) -> ("error out"=w3990:errorcluster, "State Machine out"=w3991:refnum<class "State Machine.lvclass">)  [unwired: 7 in]
                  n1438 = call-dynamic "Write State Machine.vi"("error in (no error)"=w3990, "State Machine.lvclass"=w3991, "Device in"=w3996) -> ("error out"=w3995:errorcluster, "Device out"=w3997:refnum<class "Channel.lvclass">)  [unwired: 7 in]
                  n1439 = call-dynamic "Write Channel.vi"("error in (no error)"=w3995, "Channel.lvclass"=w3997, "Acquisition in"=w3993) -> ("error out"=w4003:errorcluster, "Acquisition out"=w3992:refnum<class "Acquisition.lvclass">)  [unwired: 7 in]
                }
              }
              n1440 = call-dynamic "Write AcquisitionD.vi"("error in (no error)"=w3969, "Acquisition.lvclass"=w3965, "S4ACS_GUI in"=w3966) -> ("error out"=w3959:errorcluster, "S4ACS_GUI out"=w3960:refnum<class "S4GUI.lvclass">)  [unwired: 7 in]
            }
          }
          n1441 = Compound Arithmetic op=ADD(w3840, w3839, w3838, w3837) -> (w3836:i32)
          n1442 = case shown="0, Default" w3836 {
            tunnel: w3835 -> [w3851 _ _ _ _ _ _ _ _ _ _ _ _ _ _ _]
            tunnel: [w3850 u32 1 ("Obs_state") u32 1 ("Obs_state") u32 1 ("Obs_state") u32 1 ("Obs_state") u32 1 ("Obs_state") u32 1 ("Obs_state") u32 1 ("Obs_state") u32 1 ("Obs_state") u32 1 ("Obs_state") u32 1 ("Obs_state") u32 1 ("Obs_state") u32 1 ("Obs_state") u32 1 ("Obs_state") u32 1 ("Obs_state") u32 1 ("Obs_state")] -> w3834
            tunnel: ["" ("Error Msg") "ERROR: Lost channel 1 connection... - HandleObservationSync.vi state 325" ("Error Msg") "ERROR: Lost channel 2 connection...- HandleObservationSync.vi state 325" ("Error Msg") "ERROR: Lost channels 1 and 2 connection...- HandleObservationSync.vi state 325" ("Error Msg") "ERROR: Lost channel 3 connection...- HandleObservationSync.vi state 325" ("Error Msg") "ERROR: Lost channels 1 and  3 connection...- HandleObservationSync.vi state 325" ("Error Msg") "ERROR:  Lost channels 2 and  3 connection...- HandleObservationSync.vi state 325" ("Error Msg") "ERROR:  Lost channels 1, 2 and  3 connection...- HandleObservationSync.vi state 325" ("Error Msg") "ERROR: Lost channel 4 connection...- HandleObservationSync.vi state 325" ("Error Msg") "ERROR:  Lost channels 1 and 4 connection...- HandleObservationSync.vi state 325" ("Error Msg") "ERROR:  Lost channels 2 and 4 connection...- HandleObservationSync.vi state 325" ("Error Msg") "ERROR: Lost channels 1, 2 and 4 connection...- HandleObservationSync.vi state 325" ("Error Msg") "ERROR: Lost channels 3 and 4 connection...- HandleObservationSync.vi state 325" ("Error Msg") "ERROR: Lost channels 1, 3 and 4 connection...- HandleObservationSync.vi state 325" ("Error Msg") "ERROR: Lost channels 2, 3 and 4 connection...- HandleObservationSync.vi state 325" ("Error Msg") "ERROR: Lost channels 1, 2, 3 and 4 connection...- HandleObservationSync.vi state 325" ("Error Msg")] -> w3833
            frame 0, Default {
              n1443 = Increment(x=w3851) -> (x+1=w3850:u32)
              n1444 = Tick Count (ms)() -> (millisecond timer value=w3848:u32)
              n1445 = local write "time1"(w3848) -> ()
            }
            frame 1 {
            }
            frame 2 {
            }
            frame 3 {
            }
            frame 4 {
            }
            frame 5 {
            }
            frame 6 {
            }
            frame 7 {
            }
            frame 8 {
            }
            frame 9 {
            }
            frame 10 {
            }
            frame 11 {
            }
            frame 12 {
            }
            frame 13 {
            }
            frame 14 {
            }
            frame 15 {
            }
          }
          n1446 = Bundle By Name(cluster=w3845, "Obs_state"=w3834, "Error Msg"=w3833) -> (w3844:refnum<class "S4GUI.lvclass">)
        }
        frame 326 {
          # "Espera terminar a execução do comando atual \nantes de ir ao proximo passo da Observação."
          n1447 = call-dynamic "Read AcquisitionA.vi"("error in (no error)"=w4124, "S4ACS_GUI in"=w4125) -> ("error out"=w4106:errorcluster, "Acquisition.lvclass"=w4107:refnum<class "Acquisition.lvclass">, "S4ACS_GUI out"=w4127:refnum<class "S4GUI.lvclass">)  [unwired: 7 in]
          n1448 = call "Read connection.vi"("error in (no error)"=w4106, "Server in"=w4107) -> ("error out"=w4105:errorcluster, "connection"=w4104:bool, "Server out"=w4103:refnum<class "Acquisition.lvclass">)  [unwired: 7 in]
          n1449 = case shown="True" w4104 {
            tunnel: w4105 -> [w4223 w4244]
            tunnel: [w4224 w4242] -> w4128
            tunnel: [w4223 w4241] -> w4126
            tunnel: [TRUE w4230] -> w4085
            tunnel: w4103 -> [w4224 w4233]
            tunnel: [FALSE w4225] -> w4083
            frame False {
            }
            frame True {
              n1450 = call-dynamic "Read Channel.vi"("error in (no error)"=w4244, "Acquisition in"=w4233) -> ("error out"=w4227:errorcluster, "Channel.lvclass"=w4229:refnum<class "Channel.lvclass">, "Acquisition out"=w4243:refnum<class "Acquisition.lvclass">)  [unwired: 7 in]
              n1451 = call-dynamic "Read wait_expose.vi"("error in (no error)"=w4227, "Channel in"=w4229) -> ("error out"=w4226:errorcluster, "wait_expose"=w4225:bool, "Channel out"=w4228:refnum<class "Channel.lvclass">)  [unwired: 7 in]
              n1452 = call-dynamic "Read State Machine.vi"("error in (no error)"=w4226, "Device in"=w4228) -> ("error out"=w4235:errorcluster, "State Machine.lvclass"=w4237:refnum<class "State Machine.lvclass">, "Device out"=w4239:refnum<class "Channel.lvclass">)  [unwired: 7 in]
              n1453 = call-dynamic "Read State.vi"("error in (no error)"=w4235, "State Machine in"=w4237) -> ("error out"=w4234:errorcluster, "State"=w4231:i32, "State Machine out"=w4236:refnum<class "State Machine.lvclass">)  [unwired: 7 in]
              n1454 = Greater?(x=w4231, y=53 ("x")) -> (0:w4230:bool)
              n1455 = call-dynamic "Write State Machine.vi"("error in (no error)"=w4234, "State Machine.lvclass"=w4236, "Device in"=w4239) -> ("error out"=w4238:errorcluster, "Device out"=w4240:refnum<class "Channel.lvclass">)  [unwired: 7 in]
              n1456 = call-dynamic "Write Channel.vi"("error in (no error)"=w4238, "Channel.lvclass"=w4240, "Acquisition in"=w4243) -> ("error out"=w4241:errorcluster, "Acquisition out"=w4242:refnum<class "Acquisition.lvclass">)  [unwired: 7 in]
            }
          }
          n1457 = call-dynamic "Write AcquisitionA.vi"("error in (no error)"=w4126, "Acquisition.lvclass"=w4128, "S4ACS_GUI in"=w4127) -> ("error out"=w4121:errorcluster, "S4ACS_GUI out"=w4120:refnum<class "S4GUI.lvclass">)  [unwired: 7 in]
          n1458 = call "Read AcquisitionB.vi"("error in (no error)"=w4121, "S4ACS_GUI in"=w4120) -> ("error out"=w4098:errorcluster, "Acquisition.lvclass"=w4102:refnum<class "Acquisition.lvclass">, "S4ACS_GUI out"=w4122:refnum<class "S4GUI.lvclass">)  [unwired: 7 in]
          n1459 = call "Read connection.vi"("error in (no error)"=w4098, "Server in"=w4102) -> ("error out"=w4099:errorcluster, "connection"=w4100:bool, "Server out"=w4101:refnum<class "Acquisition.lvclass">)  [unwired: 7 in]
          n1460 = case shown="True" w4100 {
            tunnel: w4099 -> [w4199 w4212]
            tunnel: w4101 -> [w4200 w4211]
            tunnel: [TRUE w4206] -> w4087
            tunnel: [w4199 w4210] -> w4119
            tunnel: [w4200 w4209] -> w4118
            tunnel: [FALSE w4201] -> w4082
            frame False {
            }
            frame True {
              n1461 = call-dynamic "Read Channel.vi"("error in (no error)"=w4212, "Acquisition in"=w4211) -> ("error out"=w4203:errorcluster, "Channel.lvclass"=w4205:refnum<class "Channel.lvclass">, "Acquisition out"=w4213:refnum<class "Acquisition.lvclass">)  [unwired: 7 in]
              n1462 = call-dynamic "Read wait_expose.vi"("error in (no error)"=w4203, "Channel in"=w4205) -> ("error out"=w4202:errorcluster, "wait_expose"=w4201:bool, "Channel out"=w4204:refnum<class "Channel.lvclass">)  [unwired: 7 in]
              n1463 = call-dynamic "Read State Machine.vi"("error in (no error)"=w4202, "Device in"=w4204) -> ("error out"=w4219:errorcluster, "State Machine.lvclass"=w4217:refnum<class "State Machine.lvclass">, "Device out"=w4215:refnum<class "Channel.lvclass">)  [unwired: 7 in]
              n1464 = call-dynamic "Read State.vi"("error in (no error)"=w4219, "State Machine in"=w4217) -> ("error out"=w4220:errorcluster, "State"=w4208:i32, "State Machine out"=w4218:refnum<class "State Machine.lvclass">)  [unwired: 7 in]
              n1465 = Greater?(x=w4208, y=53 ("x")) -> (0:w4206:bool)
              n1466 = call-dynamic "Write State Machine.vi"("error in (no error)"=w4220, "State Machine.lvclass"=w4218, "Device in"=w4215) -> ("error out"=w4216:errorcluster, "Device out"=w4214:refnum<class "Channel.lvclass">)  [unwired: 7 in]
              n1467 = call-dynamic "Write Channel.vi"("error in (no error)"=w4216, "Channel.lvclass"=w4214, "Acquisition in"=w4213) -> ("error out"=w4210:errorcluster, "Acquisition out"=w4209:refnum<class "Acquisition.lvclass">)  [unwired: 7 in]
            }
          }
          n1468 = call "Write AcquisitionB.vi"("error in (no error)"=w4119, "Acquisition.lvclass"=w4118, "S4ACS_GUI in"=w4122) -> ("error out"=w4111:errorcluster, "S4ACS_GUI out"=w4110:refnum<class "S4GUI.lvclass">)  [unwired: 7 in]
          n1469 = call-dynamic "Read AcquisitionC.vi"("error in (no error)"=w4111, "S4ACS_GUI in"=w4110) -> ("error out"=w4094:errorcluster, "Acquisition.lvclass"=w4097:refnum<class "Acquisition.lvclass">, "S4ACS_GUI out"=w4113:refnum<class "S4GUI.lvclass">)  [unwired: 7 in]
          n1470 = call "Read connection.vi"("error in (no error)"=w4094, "Server in"=w4097) -> ("error out"=w4093:errorcluster, "connection"=w4095:bool, "Server out"=w4096:refnum<class "Acquisition.lvclass">)  [unwired: 7 in]
          n1471 = case shown="True" w4095 {
            tunnel: [w4175 w4189] -> w4114
            tunnel: [w4176 w4188] -> w4112
            tunnel: w4093 -> [w4175 w4185]
            tunnel: w4096 -> [w4176 w4186]
            tunnel: [TRUE w4182] -> w4086
            tunnel: [FALSE w4177] -> w4081
            frame False {
            }
            frame True {
              n1472 = call-dynamic "Read Channel.vi"("error in (no error)"=w4185, "Acquisition in"=w4186) -> ("error out"=w4179:errorcluster, "Channel.lvclass"=w4181:refnum<class "Channel.lvclass">, "Acquisition out"=w4187:refnum<class "Acquisition.lvclass">)  [unwired: 7 in]
              n1473 = call-dynamic "Read wait_expose.vi"("error in (no error)"=w4179, "Channel in"=w4181) -> ("error out"=w4178:errorcluster, "wait_expose"=w4177:bool, "Channel out"=w4180:refnum<class "Channel.lvclass">)  [unwired: 7 in]
              n1474 = call-dynamic "Read State Machine.vi"("error in (no error)"=w4178, "Device in"=w4180) -> ("error out"=w4195:errorcluster, "State Machine.lvclass"=w4193:refnum<class "State Machine.lvclass">, "Device out"=w4191:refnum<class "Channel.lvclass">)  [unwired: 7 in]
              n1475 = call-dynamic "Read State.vi"("error in (no error)"=w4195, "State Machine in"=w4193) -> ("error out"=w4196:errorcluster, "State"=w4183:i32, "State Machine out"=w4194:refnum<class "State Machine.lvclass">)  [unwired: 7 in]
              n1476 = Greater?(x=w4183, y=53 ("x")) -> (0:w4182:bool)
              n1477 = call-dynamic "Write State Machine.vi"("error in (no error)"=w4196, "State Machine.lvclass"=w4194, "Device in"=w4191) -> ("error out"=w4192:errorcluster, "Device out"=w4190:refnum<class "Channel.lvclass">)  [unwired: 7 in]
              n1478 = call-dynamic "Write Channel.vi"("error in (no error)"=w4192, "Channel.lvclass"=w4190, "Acquisition in"=w4187) -> ("error out"=w4189:errorcluster, "Acquisition out"=w4188:refnum<class "Acquisition.lvclass">)  [unwired: 7 in]
            }
          }
          n1479 = call-dynamic "Write AcquisitionC.vi"("error in (no error)"=w4114, "Acquisition.lvclass"=w4112, "S4ACS_GUI in"=w4113) -> ("error out"=w4108:errorcluster, "S4ACS_GUI out"=w4109:refnum<class "S4GUI.lvclass">)  [unwired: 7 in]
          n1480 = call-dynamic "Read AcquisitionD.vi"("error in (no error)"=w4108, "S4ACS_GUI in"=w4109) -> ("error out"=w4089:errorcluster, "Acquisition.lvclass"=w4092:refnum<class "Acquisition.lvclass">, "S4ACS_GUI out"=w4115:refnum<class "S4GUI.lvclass">)  [unwired: 7 in]
          n1481 = call "Read connection.vi"("error in (no error)"=w4089, "Server in"=w4092) -> ("error out"=w4088:errorcluster, "connection"=w4090:bool, "Server out"=w4091:refnum<class "Acquisition.lvclass">)  [unwired: 7 in]
          n1482 = case shown="True" w4090 {
            tunnel: [w4152 w4172] -> w4117
            tunnel: [w4151 w4171] -> w4116
            tunnel: w4091 -> [w4152 w4170]
            tunnel: w4088 -> [w4151 w4169]
            tunnel: [TRUE w4158] -> w4084
            tunnel: [FALSE w4153] -> w4080
            frame False {
            }
            frame True {
              n1483 = call-dynamic "Read Channel.vi"("error in (no error)"=w4169, "Acquisition in"=w4170) -> ("error out"=w4155:errorcluster, "Channel.lvclass"=w4157:refnum<class "Channel.lvclass">, "Acquisition out"=w4168:refnum<class "Acquisition.lvclass">)  [unwired: 7 in]
              n1484 = call-dynamic "Read wait_expose.vi"("error in (no error)"=w4155, "Channel in"=w4157) -> ("error out"=w4154:errorcluster, "wait_expose"=w4153:bool, "Channel out"=w4156:refnum<class "Channel.lvclass">)  [unwired: 7 in]
              n1485 = call-dynamic "Read State Machine.vi"("error in (no error)"=w4154, "Device in"=w4156) -> ("error out"=w4162:errorcluster, "State Machine.lvclass"=w4164:refnum<class "State Machine.lvclass">, "Device out"=w4166:refnum<class "Channel.lvclass">)  [unwired: 7 in]
              n1486 = call-dynamic "Read State.vi"("error in (no error)"=w4162, "State Machine in"=w4164) -> ("error out"=w4161:errorcluster, "State"=w4159:i32, "State Machine out"=w4163:refnum<class "State Machine.lvclass">)  [unwired: 7 in]
              n1487 = Greater?(x=w4159, y=53 ("x")) -> (0:w4158:bool)
              n1488 = call-dynamic "Write State Machine.vi"("error in (no error)"=w4161, "State Machine.lvclass"=w4163, "Device in"=w4166) -> ("error out"=w4165:errorcluster, "Device out"=w4167:refnum<class "Channel.lvclass">)  [unwired: 7 in]
              n1489 = call-dynamic "Write Channel.vi"("error in (no error)"=w4165, "Channel.lvclass"=w4167, "Acquisition in"=w4168) -> ("error out"=w4171:errorcluster, "Acquisition out"=w4172:refnum<class "Acquisition.lvclass">)  [unwired: 7 in]
            }
          }
          n1490 = call-dynamic "Write AcquisitionD.vi"("error in (no error)"=w4116, "Acquisition.lvclass"=w4117, "S4ACS_GUI in"=w4115) -> ("error out"=w4073:errorcluster, "S4ACS_GUI out"=w4075:refnum<class "S4GUI.lvclass">)  [unwired: 7 in]
          n1491 = Compound Arithmetic op=AND(w4085, w4087, w4086, w4084) -> (w4078:bool)
          n1492 = Compound Arithmetic op=OR(w4083, w4082, w4081, w4080) -> (w4079:bool)
          n1493 = call-dynamic "VerifErrors.vi"("error in (no error)"=w4073, "S4GUI in"=w4075) -> ("error out"=w4072:errorcluster, "Error value"=w4071:u32, "S4GUI out"=w4074:refnum<class "S4GUI.lvclass">)  [unwired: 7 in]
          n1494 = case shown="False" w4078 {
            tunnel: w4074 -> [w4132 w4148]
            tunnel: [w4130 w4147] -> w4076
            tunnel: w4077 -> [w4131 _]
            tunnel: w4071 -> [w4129 _]
            frame False {
              n1495 = case shown="1..15" w4129 {
                selector: w4129 -> [_ w4143]
                tunnel: [w4133 w4138] -> w4130
                tunnel: w4132 -> [w4136 w4144]
                tunnel: w4131 -> [w4135 _]
                frame 0, Default {
                  n1496 = Increment(x=w4135) -> (x+1=w4134:u32)
                  n1497 = Bundle By Name(cluster=w4136, "Obs_state"=w4134) -> (w4133:refnum<class "S4GUI.lvclass">)
                }
                frame 1..15 {
                  n1498 = Number To Decimal String(number=w4143) -> (decimal integer string=w4140:string)  [unwired: 1 in]
                  n1499 = Concatenate Strings("CHANNEL ERROR <", w4140, ">: Error flag TRUE - see ACS panel.  HandleObservationSync.vi - state 326.") -> (w4142:string)
                  n1500 = Bundle By Name(cluster=w4144, "Obs_state"=u32 1, "Error Msg"=w4142) -> (w4138:refnum<class "S4GUI.lvclass">)
                }
              }
            }
            frame True {
              # "ACTIVE detectado.\nIniciou aquisição..."
              n1501 = Tick Count (ms)() -> (millisecond timer value=w4145:u32)
              n1502 = local write "time307"(w4145) -> ()
              n1503 = Bundle By Name(cluster=w4148, "Obs_state"=u32 328) -> (w4147:refnum<class "S4GUI.lvclass">)
            }
          }
          n1504 = Bundle By Name(cluster=w4076, "mode EXPOSE"=w4079) -> (w4123:refnum<class "S4GUI.lvclass">)
        }
        frame 327 {
          # "T= canais receberam STOP"
          n1505 = Unbundle By Name(w4272) -> ("cyclesDone"=w4267:u32)
          n1506 = call-dynamic "Read AcquisitionA.vi"("error in (no error)"=w4305, "S4ACS_GUI in"=w4272) -> ("error out"=w4287:errorcluster, "Acquisition.lvclass"=w4288:refnum<class "Acquisition.lvclass">, "S4ACS_GUI out"=w4307:refnum<class "S4GUI.lvclass">)  [unwired: 7 in]
          n1507 = call-dynamic "Read enabled.vi"("error in (no error)"=w4287, "Server in"=w4288) -> ("error out"=w4286:errorcluster, "enabled"=w4263:bool, "Server out"=w4285:refnum<class "Acquisition.lvclass">)  [unwired: 7 in]
          n1508 = case shown="True" w4263 {
            tunnel: w4286 -> [w4458 w4475]
            tunnel: [w4459 w4473] -> w4308
            tunnel: [w4458 w4472] -> w4306
            tunnel: [0 ("State") w4468] -> w4258
            tunnel: w4285 -> [w4459 w4467]
            tunnel: w4267 -> [_ w4466]
            tunnel: [TRUE w4465] -> w4271
            tunnel: [FALSE ("stopping") w4461] -> w4254
            frame False {
            }
            frame True {
              n1509 = call-dynamic "Read Channel.vi"("error in (no error)"=w4475, "Acquisition in"=w4467) -> ("error out"=w4471:errorcluster, "Channel.lvclass"=w4470:refnum<class "Channel.lvclass">, "Acquisition out"=w4474:refnum<class "Acquisition.lvclass">)  [unwired: 7 in]
              n1510 = call-dynamic "Read CyclesDone.vi"("error in (no error)"=w4471, "Channel in"=w4470) -> ("error out"=w4463:errorcluster, "CyclesDone"=w4468:u32, "Channel out"=w4469:refnum<class "Channel.lvclass">)  [unwired: 7 in]
              n1511 = Increment(x=w4466) -> (x+1=w4460:u32)
              n1512 = Equal?(x=w4468, y=w4460) -> (x = y?=w4465:bool)
              n1513 = call-dynamic "Read stopping.vi"("error in (no error)"=w4463, "Channel in"=w4469) -> ("error out"=w4462:errorcluster, "stopping"=w4461:bool, "Channel out"=w4464:refnum<class "Channel.lvclass">)  [unwired: 7 in]
              n1514 = call-dynamic "Write Channel.vi"("error in (no error)"=w4462, "Channel.lvclass"=w4464, "Acquisition in"=w4474) -> ("error out"=w4472:errorcluster, "Acquisition out"=w4473:refnum<class "Acquisition.lvclass">)  [unwired: 7 in]
            }
          }
